vi "Set Style.vi"(8 "error in (no error)":errorcluster, 10 "Styles.lvlib:Style.lvclass":refnum<class "Style.lvclass">, 11 "xwpfRun in":refnum<class "xwpfRun.lvclass">) -> (0 "error out":errorcluster, 3 "xwpfRun out":refnum<class "xwpfRun.lvclass">)   [LabVIEW 2017, in "Word_Specific.lvlib" / "xwpfRun.lvclass"]
uses:
  xwpfRun.lvclass
  Styles/Style/Style.lvclass
  xwpfRun.lvclass/xwpfRun.ctl
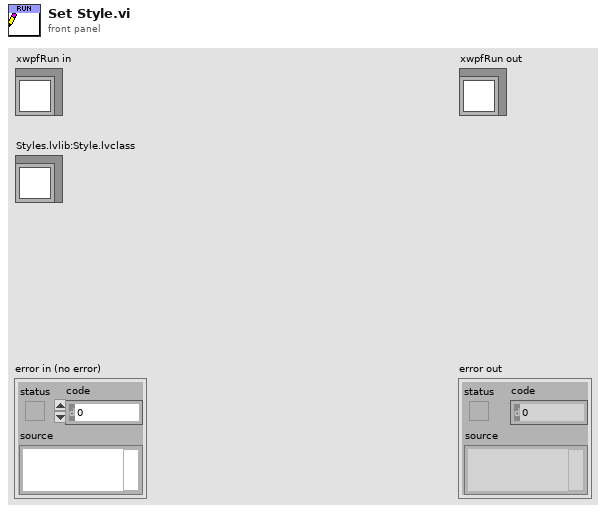
[diagram p1: front panel]
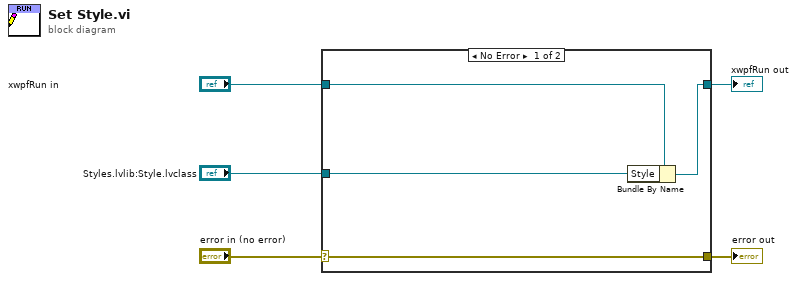
[diagram p0: block diagram]
diagram:
  n1 = case shown="No Error" "error in (no error)" {
    selector: "error in (no error)" -> [w9 w10]
    tunnel: [w9 w10] -> w4
    tunnel: [w7 w11] -> w2
    tunnel: "xwpfRun in" -> [w8 w11]
    tunnel: "Styles.lvlib:Style.lvclass" -> [w6 _]
    frame No Error {
      n2 = Bundle By Name(cluster=w8, "Style"=w6) -> (w7:refnum<class "xwpfRun.lvclass">)
    }
    frame Error {
    }
  }
  "error out" <- w4
  "xwpfRun out" <- w2
